vi "fgv_DS1202_usb.vi"(7 "cmd":T1, 8 "error in":errorcluster) -> (0 "error out":errorcluster, 3 "wfm":waveform(dbl)(graph))   [LabVIEW 2021]
uses:
  ctrl/DS1202_cmd.ctl
  ctrl/rw.ctl
  ctrl/instr-hw.ctl
  <instrlib>/RIGOL DS1000 Series/Public/Data/Read (Single Waveform).vi
  <instrlib>/RIGOL DS1000 Series/RIGOL DS1000 Series.lvlib
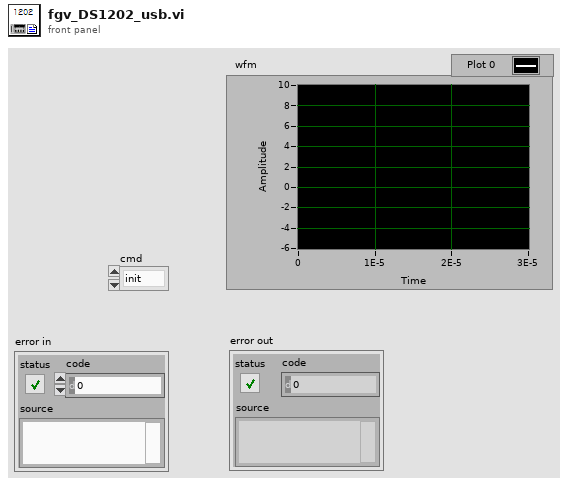
[diagram p1: front panel]
types:
  T1 = typedef "DS1202_cmd.ctl" = enum16{"init", "auto", "read", "close"}
  T2 = typedef "rw.ctl" = enum16{"read", "write"}
  T3 = typedef "DS1202_cfg.ctl" = cluster{"VISA ":refnum<visa-resource-name>, "Timeout":u32, "Channel":u16}
  T4 = typedef "instr-hw.ctl" = enum16{"PXIe-5110", "PXIe-5431", "PXIe-2530", "DS1202"}
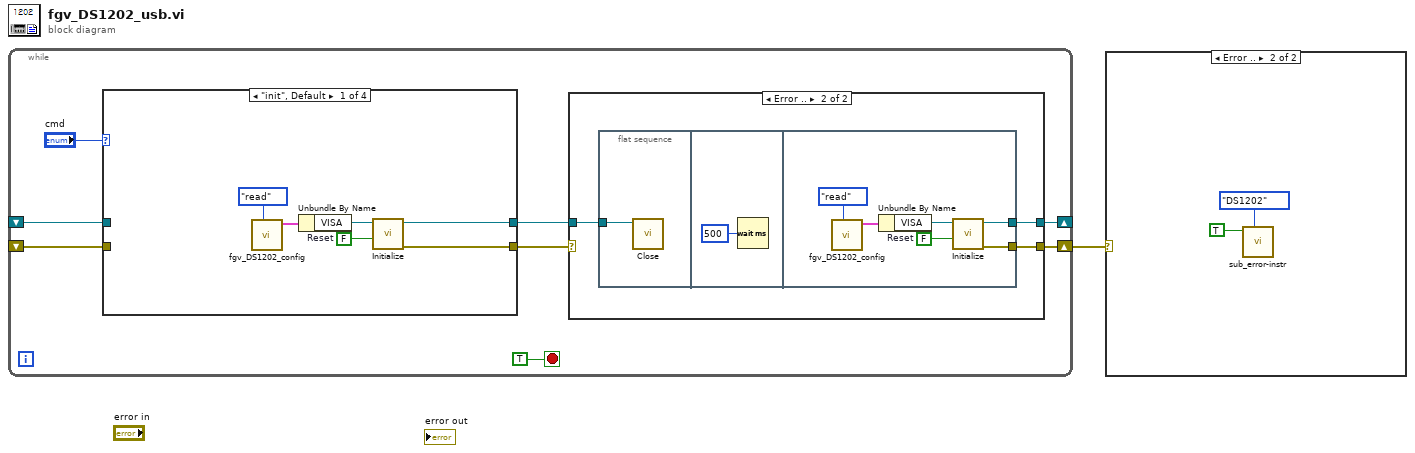
[diagram p0: block diagram]
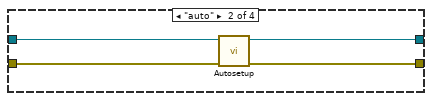
[diagram p4: hidden frame]
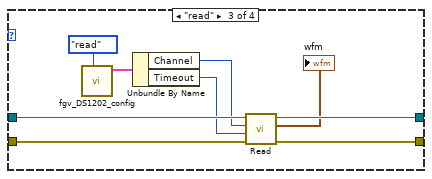
[diagram p5: hidden frame]
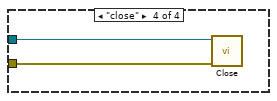
[diagram p6: hidden frame]
diagram:
  n1 = while {
    shift-right: [w4] -> _
    shift-left: _ -> [w7]
    shift-right: [w2] -> w1
    shift-left: _ -> [w6]
    stop <- TRUE stop-if-true
    n2 = case shown="\"init\", Default" "cmd" {
      tunnel: [w27 w29 w40 _] -> w3
      tunnel: [w26 w30 w41 _] -> w5
      tunnel: w7 -> [_ w32 w39 w42]
      tunnel: w6 -> [_ w31 w38 w43]
      frame "init", Default {
        w28 = FALSE  # Reset
        n3 = call "fgv_DS1202_config.vi"("cmd"=rw."read") -> ("config 2"=w24:T3)  [unwired: 10 in]
        n4 = Unbundle By Name(w24) -> ("VISA"=w23:refnum<visa-resource-name>)
        n5 = call <instrlib>:"Initialize.vi"("Reset (True)"=w28, "VISA resource name"=w23) -> ("error out"=w26:errorcluster, "VISA resource name out"=w27:refnum<visa-resource-name>)  [unwired: 2 in, 6 out]
      }
      frame "auto" {
        n6 = call <instrlib>:"Autosetup.vi"("error in (no error)"=w31, "VISA resource name"=w32) -> ("error out"=w30:errorcluster, "VISA resource name out"=w29:refnum<visa-resource-name>)  [unwired: 8 out]
      }
      frame "read" {
        n7 = call "fgv_DS1202_config.vi"("cmd"=rw."read") -> ("config 2"=w36:T3)  [unwired: 10 in]
        n8 = Unbundle By Name(w36) -> ("Channel"=w35:u16, "Timeout"=w34:u32)
        n9 = call-poly <instrlib>:"Read.vi"("error in (no error)"=w38, "Timeout (10000 ms)"=w34, "Channel (0: Channel 1)"=w35, "VISA resource name"=w39) -> ("error out"=w41:errorcluster, "Waveform Data"=→"wfm":waveform(dbl), "VISA resource name out"=w40:refnum<visa-resource-name>)  [unwired: 5 out]
      }
      frame "close" {
        n10 = call <instrlib>:"Close.vi"("error in (no error)"=w43, "VISA resource name"=w42) -> ()  [unwired: 10 out]
      }
    }
    n11 = case shown="Error .." w5 {
      selector: w5 -> [w10 _]
      tunnel: [w11 w12] -> w4
      tunnel: w3 -> [w11 w14]
      tunnel: [w10 w13] -> w2
      frame No Error {
      }
      frame Error {
        n12 = flat-sequence {
          tunnel: w14 -> [w15]
          tunnel: [w18] -> w13
          tunnel: [w17] -> w12
          frame #0 {
            n13 = call <instrlib>:"Close.vi"("VISA resource name"=w15) -> ()  [unwired: 1 in, 10 out]
          }
          frame #1 {
            n14 = Wait (ms)(milliseconds to wait=u32 500) -> ()  [unwired: 1 out]
          }
          frame #2 {
            w19 = FALSE  # Reset
            n15 = call "fgv_DS1202_config.vi"("cmd"=rw."read") -> ("config 2"=w21:T3)  [unwired: 10 in]
            n16 = Unbundle By Name(w21) -> ("VISA"=w22:refnum<visa-resource-name>)
            n17 = call <instrlib>:"Initialize.vi"("Reset (True)"=w19, "VISA resource name"=w22) -> ("error out"=w18:errorcluster, "VISA resource name out"=w17:refnum<visa-resource-name>)  [unwired: 2 in, 6 out]
          }
        }
      }
    }
  }
  n18 = case shown="Error .." w1 {
    frame No Error {
    }
    frame Error {
      n19 = call "sub_error-instr.vi"("instr sel"=instr-hw."DS1202", "error"=TRUE) -> ()  [unwired: 10 in]
    }
  }
